vi "UIRef.vi"(8 "error in":errorcluster, 11 "node in":refnum<class "Targets.lvclass">) -> (0 "error out":errorcluster, 2 "VI refnum":refnum<vi>, 3 "node out":refnum<class "Targets.lvclass">)   [LabVIEW 2015, in "Targets.lvclass"]
doc: "Stores the static reference to the UI of the node."
uses:
  Targets.lvclass
  TargetsUI.vi
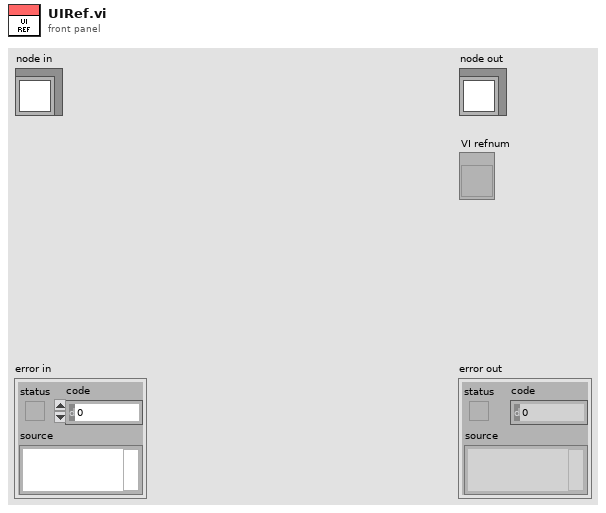
[diagram p1: front panel]
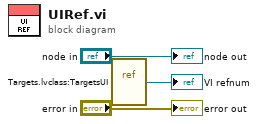
[diagram p0: block diagram]
diagram:
  n1 = vi-ref "Targets.lvclass:TargetsUI.vi"() -> (→"VI refnum":refnum<vi>)
  "error out" <- "error in"
  "node out" <- "node in"
